vi "Determine Sector Edge Location.vi"() -> (0 "Prev Right Sect":u8, 1 "Prev Left Sect":u8, 2 "Left Sector Edge":u8, 3 "Right Sector Edge":u8)   [LabVIEW 2013]
doc: "Takes the average sector intensities and compares each average to the threshold value to determine which sector the edge is located in."
uses:
  Globals/Accumulated Sector Intensity.vi
  Globals/Sector Parameter Global.vi
  <vilib>/rvi/FIFO/Fifo_Resource/nirvififoEmulationReadFpgaImpl.vi
  <vilib>/rvi/DataTransferAndStorage/Container/Common/niFpgaContainerGetUniqueNameForEmu.vi
  <vilib>/rvi/interface/RandomDataEmulation/nirviRandomDataFPGAFIFO.vi
  <vilib>/rvi/interface/RandomDataEmulation/niFpgaRandomDataHandleErrors.vi
  <vilib>/rvi/DataTransferAndStorage/Container/XNode/niFpgaContainer.xnode
  <vilib>/rvi/FIFO/Fifo_Resource/nirvififoEmulationRead.vi
  <vilib>/rvi/interface/RandomDataEmulation/nirviRandomDataFpgaReadWriteTemplate.vi
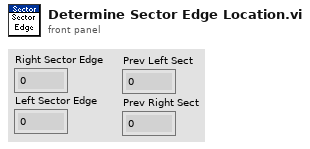
[diagram p1: front panel]
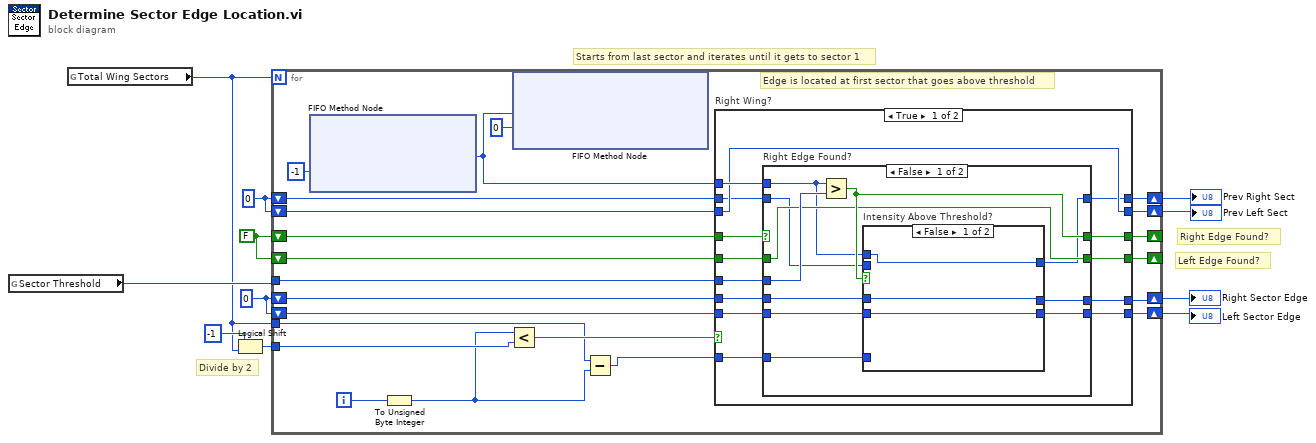
[diagram p0: block diagram]
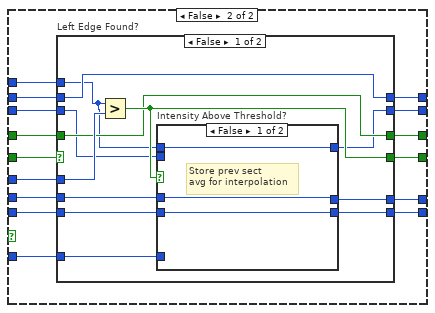
[diagram p4: hidden frame]
diagram:
  w3 = u8 0 ("Total Wing Sectors")
  w6 = u8 0 ("Total Wing Sectors")
  w7 = FALSE ("Left Edge Found?")
  # "Starts from last sector and iterates until it gets to sector 1"
  # "Left Edge Found?"
  # "Right Edge Found?"
  # "Divide by 2"
  n1 = global read "Sector Parameter Global.vi" "Sector Threshold"() -> (w5:u8)
  n2 = global read "Accumulated Sector Intensity.vi" "Total Wing Sectors"() -> (w4:u8)
  n3 = Logical Shift(y=i16 -1, x=w4) -> (x << y=w8:u8)
  n4 = for {
    N: w4 -> [_]
    tunnel: w5 -> [w31]
    tunnel: w8 -> [w32]
    shift-right: [w29] -> _
    shift-left: w7 -> [w30]
    shift-right: [w22] -> _
    shift-left: w7 -> [w23]
    shift-right: [w27] -> w11
    shift-left: w6 -> [w26]
    shift-right: [w25] -> w10
    shift-left: w6 -> [w24]
    tunnel: w4 -> [w18]
    shift-right: [w13] -> w2
    shift-left: w3 -> [w12]
    shift-right: [w14] -> w1
    shift-left: w3 -> [w15]
    i -> [w28]
    # "Edge is located at first sector that goes above threshold"
    n5 = xnode ("FIFO Method Node")("Timeout"=-1) -> ("Element"=w21:u8)  [unwired: 1 in, 2 out]
    n6 = To Unsigned Byte Integer(number=w28) -> (unsigned 8bit integer=w17:u8)
    n7 = Less?(x=w17, y=w32) -> (x < y?=w33:bool)
    n8 = xnode ("FIFO Method Node")("Element"=w21, "Timeout"=0) -> ()  [unwired: 1 in, 2 out]
    n9 = Subtract(x=w18, y=w17) -> (x-y=w16:u8)
    n10 = case "Right Wing?" shown="True" w33 {
      tunnel: w21 -> [w46 w84]
      tunnel: w31 -> [w45 w83]
      tunnel: w30 -> [w47 w75]
      tunnel: [w44 w82] -> w29
      tunnel: w16 -> [w43 w81]
      tunnel: [w42 w80] -> w27
      tunnel: w26 -> [w41 w79]
      tunnel: [w40 w78] -> w25
      tunnel: w24 -> [w39 w77]
      tunnel: w23 -> [w38 w76]
      tunnel: [w37 w74] -> w22
      tunnel: w15 -> [w36 w73]
      tunnel: [w36 w72] -> w14
      tunnel: [w34 w71] -> w13
      tunnel: w12 -> [w35 w70]
      frame True {
        n11 = case "Right Edge Found?" shown="False" w47 {
          selector: w47 -> [_ w66]
          tunnel: w46 -> [w50 _]
          tunnel: w45 -> [w58 _]
          tunnel: [w57 w66] -> w44
          tunnel: w43 -> [w56 _]
          tunnel: [w55 w69] -> w42
          tunnel: w41 -> [w54 w69]
          tunnel: [w53 w68] -> w40
          tunnel: w39 -> [w52 w68]
          tunnel: w38 -> [w51 w67]
          tunnel: [w51 w67] -> w37
          tunnel: w35 -> [w48 w65]
          tunnel: [w49 w65] -> w34
          frame False {
            n12 = Greater?(x=w50, y=w58) -> (0:w57:bool)
            n13 = case "Intensity Above Threshold?" shown="False" w57 {
              tunnel: w56 -> [_ w63]
              tunnel: [w61 w63] -> w55
              tunnel: w54 -> [w61 _]
              tunnel: [w60 w64] -> w53
              tunnel: w52 -> [w60 w64]
              tunnel: w50 -> [w59 _]
              tunnel: [w59 w62] -> w49
              tunnel: w48 -> [_ w62]
              frame False {
              }
              frame True {
              }
            }
          }
          frame True {
          }
        }
      }
      frame False {
        n14 = case "Left Edge Found?" shown="False" w76 {
          selector: w76 -> [_ w105]
          tunnel: w84 -> [w85 _]
          tunnel: w83 -> [w96 _]
          tunnel: [w89 w106] -> w82
          tunnel: w81 -> [w95 _]
          tunnel: [w94 w108] -> w80
          tunnel: w79 -> [w93 w108]
          tunnel: [w92 w107] -> w78
          tunnel: w77 -> [w91 w107]
          tunnel: w75 -> [w89 w106]
          tunnel: [w90 w105] -> w74
          tunnel: w73 -> [w88 w104]
          tunnel: [w87 w104] -> w72
          tunnel: [w86 w103] -> w71
          tunnel: w70 -> [w86 w103]
          frame False {
            n15 = Greater?(x=w85, y=w96) -> (0:w90:bool)
            n16 = case "Intensity Above Threshold?" shown="False" w90 {
              tunnel: w95 -> [_ w101]
              tunnel: [w99 w102] -> w94
              tunnel: w93 -> [w99 w102]
              tunnel: [w98 w101] -> w92
              tunnel: w91 -> [w98 _]
              tunnel: w88 -> [_ w100]
              tunnel: [w97 w100] -> w87
              tunnel: w85 -> [w97 _]
              frame False {
                # "Store prev sect\navg for interpolation"
              }
              frame True {
              }
            }
          }
          frame True {
          }
        }
      }
    }
  }
  "Right Sector Edge" <- w11
  "Left Sector Edge" <- w10
  "Prev Right Sect" <- w2
  "Prev Left Sect" <- w1
